vi "波形记录处理.vi"(8 "控件配置文件":string[][](table), 9 "表格":string[][](table)) -> (0 "曲线数量":u16, 2 "曲线名称":string[](array[string]), 3 "波形图":dynamicdata(graph))   [LabVIEW 2021]
uses:
  controls/DataInitDef.ctl
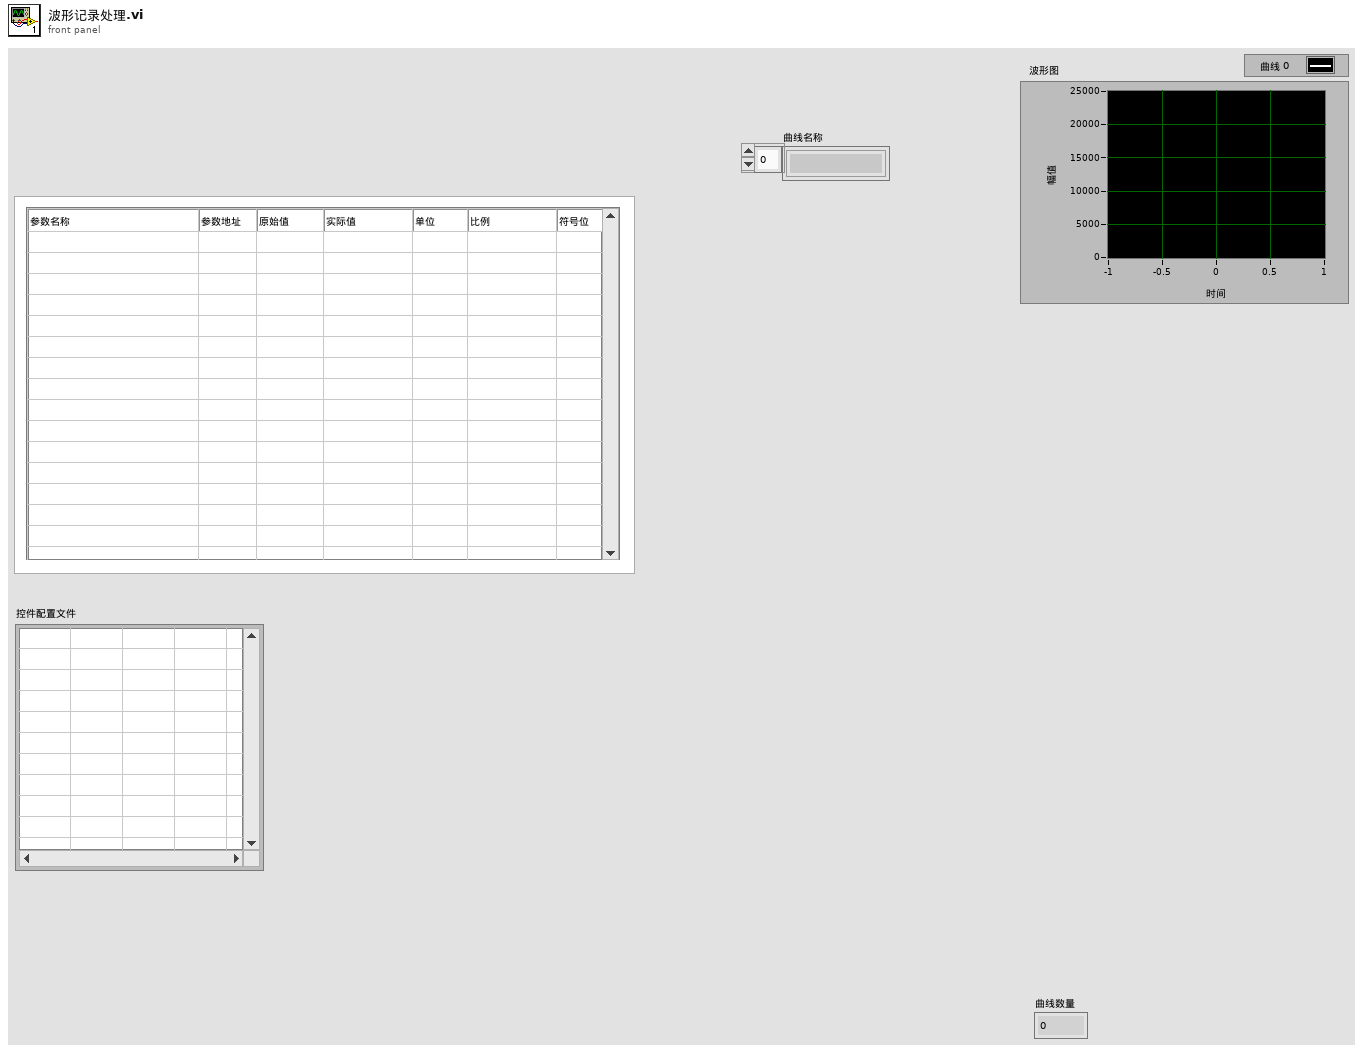
[diagram p1: front panel]
types:
  T1 = typedef "DataInitDef.ctl" = u16
  T2 = cluster{"显示":string, "显示":string, "显示":string, "显示":string, "显示":string, "显示":string, "显示":string, "显示":string, "显示":string, "显示":string, "显示":string, "显示":string, "显示":string, "显示":string, "显示":string, "显示":string}
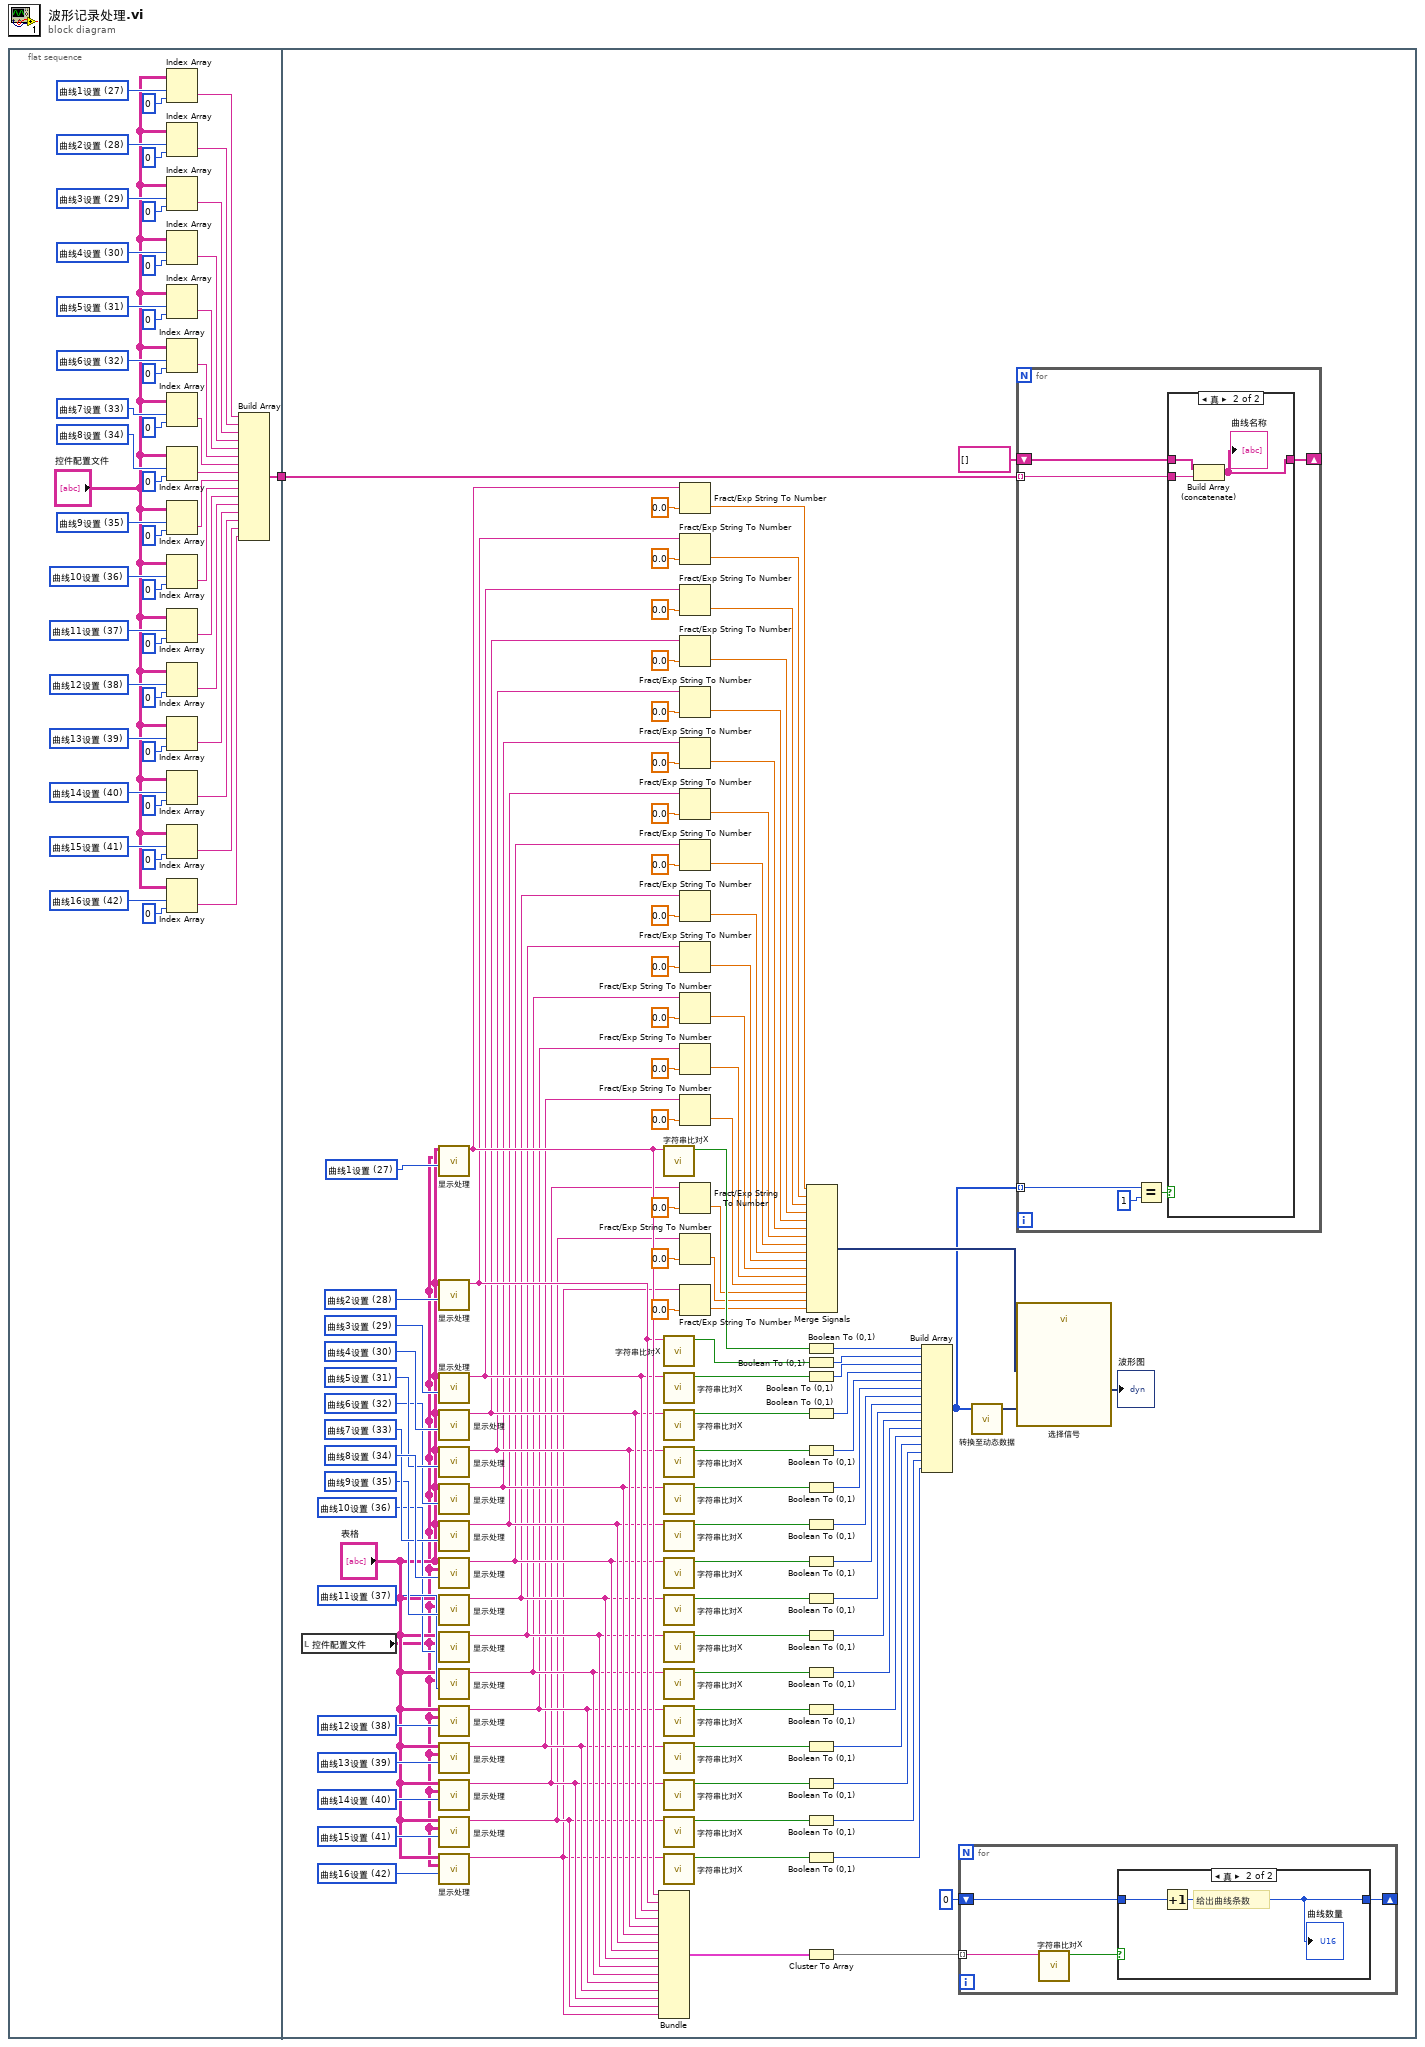
[diagram p0: block diagram]
diagram:
  n1 = flat-sequence {
    tunnel: [w27] -> w1
    tunnel: w1 -> [w115]
    frame #0 {
      w26 = T1 42 items=["刷新间隔", "波特率", "布尔1设置项", "布尔2设置项", "布尔3设置项", "布尔4设置项", "布尔5设置项", "显控1设置", "显控2设置", "显控3设置", "显控4设置", "显控5设置", "显控6设置", "显控7设置", "显控8设置", "显控9设置", "显控10设置", "显控11设置", "显控12设置", "设控1设置", "设控2设置", "设控3设置", "设控4设置", "设控5设置", "设控6设置", "设控7设置", "设控8设置", "曲线1设置", "曲线2设置", "曲线3设置", "曲线4设置", "曲线5设置", "曲线6设置", "曲线7设置", "曲线8设置", "曲线9设置", "曲线10设置", "曲线11设置", "曲线12设置", "曲线13设置", "曲线14设置", "曲线15设置", "曲线16设置", "ID值"] ("DataInitDef")
      w24 = T1 41 items=["刷新间隔", "波特率", "布尔1设置项", "布尔2设置项", "布尔3设置项", "布尔4设置项", "布尔5设置项", "显控1设置", "显控2设置", "显控3设置", "显控4设置", "显控5设置", "显控6设置", "显控7设置", "显控8设置", "显控9设置", "显控10设置", "显控11设置", "显控12设置", "设控1设置", "设控2设置", "设控3设置", "设控4设置", "设控5设置", "设控6设置", "设控7设置", "设控8设置", "曲线1设置", "曲线2设置", "曲线3设置", "曲线4设置", "曲线5设置", "曲线6设置", "曲线7设置", "曲线8设置", "曲线9设置", "曲线10设置", "曲线11设置", "曲线12设置", "曲线13设置", "曲线14设置", "曲线15设置", "曲线16设置", "ID值"] ("DataInitDef")
      w22 = T1 40 items=["刷新间隔", "波特率", "布尔1设置项", "布尔2设置项", "布尔3设置项", "布尔4设置项", "布尔5设置项", "显控1设置", "显控2设置", "显控3设置", "显控4设置", "显控5设置", "显控6设置", "显控7设置", "显控8设置", "显控9设置", "显控10设置", "显控11设置", "显控12设置", "设控1设置", "设控2设置", "设控3设置", "设控4设置", "设控5设置", "设控6设置", "设控7设置", "设控8设置", "曲线1设置", "曲线2设置", "曲线3设置", "曲线4设置", "曲线5设置", "曲线6设置", "曲线7设置", "曲线8设置", "曲线9设置", "曲线10设置", "曲线11设置", "曲线12设置", "曲线13设置", "曲线14设置", "曲线15设置", "曲线16设置", "ID值"] ("DataInitDef")
      w20 = T1 39 items=["刷新间隔", "波特率", "布尔1设置项", "布尔2设置项", "布尔3设置项", "布尔4设置项", "布尔5设置项", "显控1设置", "显控2设置", "显控3设置", "显控4设置", "显控5设置", "显控6设置", "显控7设置", "显控8设置", "显控9设置", "显控10设置", "显控11设置", "显控12设置", "设控1设置", "设控2设置", "设控3设置", "设控4设置", "设控5设置", "设控6设置", "设控7设置", "设控8设置", "曲线1设置", "曲线2设置", "曲线3设置", "曲线4设置", "曲线5设置", "曲线6设置", "曲线7设置", "曲线8设置", "曲线9设置", "曲线10设置", "曲线11设置", "曲线12设置", "曲线13设置", "曲线14设置", "曲线15设置", "曲线16设置", "ID值"] ("DataInitDef")
      w18 = T1 38 items=["刷新间隔", "波特率", "布尔1设置项", "布尔2设置项", "布尔3设置项", "布尔4设置项", "布尔5设置项", "显控1设置", "显控2设置", "显控3设置", "显控4设置", "显控5设置", "显控6设置", "显控7设置", "显控8设置", "显控9设置", "显控10设置", "显控11设置", "显控12设置", "设控1设置", "设控2设置", "设控3设置", "设控4设置", "设控5设置", "设控6设置", "设控7设置", "设控8设置", "曲线1设置", "曲线2设置", "曲线3设置", "曲线4设置", "曲线5设置", "曲线6设置", "曲线7设置", "曲线8设置", "曲线9设置", "曲线10设置", "曲线11设置", "曲线12设置", "曲线13设置", "曲线14设置", "曲线15设置", "曲线16设置", "ID值"] ("DataInitDef")
      w16 = T1 37 items=["刷新间隔", "波特率", "布尔1设置项", "布尔2设置项", "布尔3设置项", "布尔4设置项", "布尔5设置项", "显控1设置", "显控2设置", "显控3设置", "显控4设置", "显控5设置", "显控6设置", "显控7设置", "显控8设置", "显控9设置", "显控10设置", "显控11设置", "显控12设置", "设控1设置", "设控2设置", "设控3设置", "设控4设置", "设控5设置", "设控6设置", "设控7设置", "设控8设置", "曲线1设置", "曲线2设置", "曲线3设置", "曲线4设置", "曲线5设置", "曲线6设置", "曲线7设置", "曲线8设置", "曲线9设置", "曲线10设置", "曲线11设置", "曲线12设置", "曲线13设置", "曲线14设置", "曲线15设置", "曲线16设置", "ID值"] ("DataInitDef")
      w14 = T1 36 items=["刷新间隔", "波特率", "布尔1设置项", "布尔2设置项", "布尔3设置项", "布尔4设置项", "布尔5设置项", "显控1设置", "显控2设置", "显控3设置", "显控4设置", "显控5设置", "显控6设置", "显控7设置", "显控8设置", "显控9设置", "显控10设置", "显控11设置", "显控12设置", "设控1设置", "设控2设置", "设控3设置", "设控4设置", "设控5设置", "设控6设置", "设控7设置", "设控8设置", "曲线1设置", "曲线2设置", "曲线3设置", "曲线4设置", "曲线5设置", "曲线6设置", "曲线7设置", "曲线8设置", "曲线9设置", "曲线10设置", "曲线11设置", "曲线12设置", "曲线13设置", "曲线14设置", "曲线15设置", "曲线16设置", "ID值"] ("DataInitDef")
      w12 = T1 35 items=["刷新间隔", "波特率", "布尔1设置项", "布尔2设置项", "布尔3设置项", "布尔4设置项", "布尔5设置项", "显控1设置", "显控2设置", "显控3设置", "显控4设置", "显控5设置", "显控6设置", "显控7设置", "显控8设置", "显控9设置", "显控10设置", "显控11设置", "显控12设置", "设控1设置", "设控2设置", "设控3设置", "设控4设置", "设控5设置", "设控6设置", "设控7设置", "设控8设置", "曲线1设置", "曲线2设置", "曲线3设置", "曲线4设置", "曲线5设置", "曲线6设置", "曲线7设置", "曲线8设置", "曲线9设置", "曲线10设置", "曲线11设置", "曲线12设置", "曲线13设置", "曲线14设置", "曲线15设置", "曲线16设置", "ID值"] ("DataInitDef")
      w51 = T1 34 items=["刷新间隔", "波特率", "布尔1设置项", "布尔2设置项", "布尔3设置项", "布尔4设置项", "布尔5设置项", "显控1设置", "显控2设置", "显控3设置", "显控4设置", "显控5设置", "显控6设置", "显控7设置", "显控8设置", "显控9设置", "显控10设置", "显控11设置", "显控12设置", "设控1设置", "设控2设置", "设控3设置", "设控4设置", "设控5设置", "设控6设置", "设控7设置", "设控8设置", "曲线1设置", "曲线2设置", "曲线3设置", "曲线4设置", "曲线5设置", "曲线6设置", "曲线7设置", "曲线8设置", "曲线9设置", "曲线10设置", "曲线11设置", "曲线12设置", "曲线13设置", "曲线14设置", "曲线15设置", "曲线16设置", "ID值"] ("DataInitDef")
      w49 = T1 33 items=["刷新间隔", "波特率", "布尔1设置项", "布尔2设置项", "布尔3设置项", "布尔4设置项", "布尔5设置项", "显控1设置", "显控2设置", "显控3设置", "显控4设置", "显控5设置", "显控6设置", "显控7设置", "显控8设置", "显控9设置", "显控10设置", "显控11设置", "显控12设置", "设控1设置", "设控2设置", "设控3设置", "设控4设置", "设控5设置", "设控6设置", "设控7设置", "设控8设置", "曲线1设置", "曲线2设置", "曲线3设置", "曲线4设置", "曲线5设置", "曲线6设置", "曲线7设置", "曲线8设置", "曲线9设置", "曲线10设置", "曲线11设置", "曲线12设置", "曲线13设置", "曲线14设置", "曲线15设置", "曲线16设置", "ID值"] ("DataInitDef")
      w47 = T1 32 items=["刷新间隔", "波特率", "布尔1设置项", "布尔2设置项", "布尔3设置项", "布尔4设置项", "布尔5设置项", "显控1设置", "显控2设置", "显控3设置", "显控4设置", "显控5设置", "显控6设置", "显控7设置", "显控8设置", "显控9设置", "显控10设置", "显控11设置", "显控12设置", "设控1设置", "设控2设置", "设控3设置", "设控4设置", "设控5设置", "设控6设置", "设控7设置", "设控8设置", "曲线1设置", "曲线2设置", "曲线3设置", "曲线4设置", "曲线5设置", "曲线6设置", "曲线7设置", "曲线8设置", "曲线9设置", "曲线10设置", "曲线11设置", "曲线12设置", "曲线13设置", "曲线14设置", "曲线15设置", "曲线16设置", "ID值"] ("DataInitDef")
      w45 = T1 31 items=["刷新间隔", "波特率", "布尔1设置项", "布尔2设置项", "布尔3设置项", "布尔4设置项", "布尔5设置项", "显控1设置", "显控2设置", "显控3设置", "显控4设置", "显控5设置", "显控6设置", "显控7设置", "显控8设置", "显控9设置", "显控10设置", "显控11设置", "显控12设置", "设控1设置", "设控2设置", "设控3设置", "设控4设置", "设控5设置", "设控6设置", "设控7设置", "设控8设置", "曲线1设置", "曲线2设置", "曲线3设置", "曲线4设置", "曲线5设置", "曲线6设置", "曲线7设置", "曲线8设置", "曲线9设置", "曲线10设置", "曲线11设置", "曲线12设置", "曲线13设置", "曲线14设置", "曲线15设置", "曲线16设置", "ID值"] ("DataInitDef")
      w43 = T1 30 items=["刷新间隔", "波特率", "布尔1设置项", "布尔2设置项", "布尔3设置项", "布尔4设置项", "布尔5设置项", "显控1设置", "显控2设置", "显控3设置", "显控4设置", "显控5设置", "显控6设置", "显控7设置", "显控8设置", "显控9设置", "显控10设置", "显控11设置", "显控12设置", "设控1设置", "设控2设置", "设控3设置", "设控4设置", "设控5设置", "设控6设置", "设控7设置", "设控8设置", "曲线1设置", "曲线2设置", "曲线3设置", "曲线4设置", "曲线5设置", "曲线6设置", "曲线7设置", "曲线8设置", "曲线9设置", "曲线10设置", "曲线11设置", "曲线12设置", "曲线13设置", "曲线14设置", "曲线15设置", "曲线16设置", "ID值"] ("DataInitDef")
      w41 = T1 29 items=["刷新间隔", "波特率", "布尔1设置项", "布尔2设置项", "布尔3设置项", "布尔4设置项", "布尔5设置项", "显控1设置", "显控2设置", "显控3设置", "显控4设置", "显控5设置", "显控6设置", "显控7设置", "显控8设置", "显控9设置", "显控10设置", "显控11设置", "显控12设置", "设控1设置", "设控2设置", "设控3设置", "设控4设置", "设控5设置", "设控6设置", "设控7设置", "设控8设置", "曲线1设置", "曲线2设置", "曲线3设置", "曲线4设置", "曲线5设置", "曲线6设置", "曲线7设置", "曲线8设置", "曲线9设置", "曲线10设置", "曲线11设置", "曲线12设置", "曲线13设置", "曲线14设置", "曲线15设置", "曲线16设置", "ID值"] ("DataInitDef")
      w39 = T1 28 items=["刷新间隔", "波特率", "布尔1设置项", "布尔2设置项", "布尔3设置项", "布尔4设置项", "布尔5设置项", "显控1设置", "显控2设置", "显控3设置", "显控4设置", "显控5设置", "显控6设置", "显控7设置", "显控8设置", "显控9设置", "显控10设置", "显控11设置", "显控12设置", "设控1设置", "设控2设置", "设控3设置", "设控4设置", "设控5设置", "设控6设置", "设控7设置", "设控8设置", "曲线1设置", "曲线2设置", "曲线3设置", "曲线4设置", "曲线5设置", "曲线6设置", "曲线7设置", "曲线8设置", "曲线9设置", "曲线10设置", "曲线11设置", "曲线12设置", "曲线13设置", "曲线14设置", "曲线15设置", "曲线16设置", "ID值"] ("DataInitDef")
      w37 = T1 27 items=["刷新间隔", "波特率", "布尔1设置项", "布尔2设置项", "布尔3设置项", "布尔4设置项", "布尔5设置项", "显控1设置", "显控2设置", "显控3设置", "显控4设置", "显控5设置", "显控6设置", "显控7设置", "显控8设置", "显控9设置", "显控10设置", "显控11设置", "显控12设置", "设控1设置", "设控2设置", "设控3设置", "设控4设置", "设控5设置", "设控6设置", "设控7设置", "设控8设置", "曲线1设置", "曲线2设置", "曲线3设置", "曲线4设置", "曲线5设置", "曲线6设置", "曲线7设置", "曲线8设置", "曲线9设置", "曲线10设置", "曲线11设置", "曲线12设置", "曲线13设置", "曲线14设置", "曲线15设置", "曲线16设置", "ID值"] ("DataInitDef")
      n2 = Index Array(array="控件配置文件", index (row)=w37, index (col)=0 ("禁用的索引 (列)")) -> (element=w35:string)
      n3 = Index Array(array="控件配置文件", index (row)=w39, index (col)=0 ("禁用的索引 (列)")) -> (element=w34:string)
      n4 = Index Array(array="控件配置文件", index (row)=w41, index (col)=0 ("禁用的索引 (列)")) -> (element=w33:string)
      n5 = Index Array(array="控件配置文件", index (row)=w43, index (col)=0 ("禁用的索引 (列)")) -> (element=w32:string)
      n6 = Index Array(array="控件配置文件", index (row)=w45, index (col)=0 ("禁用的索引 (列)")) -> (element=w31:string)
      n7 = Index Array(array="控件配置文件", index (row)=w47, index (col)=0 ("禁用的索引 (列)")) -> (element=w30:string)
      n8 = Index Array(array="控件配置文件", index (row)=w49, index (col)=0 ("禁用的索引 (列)")) -> (element=w28:string)
      n9 = Index Array(array="控件配置文件", index (row)=w51, index (col)=0 ("禁用的索引 (列)")) -> (element=w29:string)
      n10 = Index Array(array="控件配置文件", index (row)=w12, index (col)=0 ("禁用的索引 (列)")) -> (element=w9:string)
      n11 = Index Array(array="控件配置文件", index (row)=w14, index (col)=0 ("禁用的索引 (列)")) -> (element=w8:string)
      n12 = Index Array(array="控件配置文件", index (row)=w16, index (col)=0 ("禁用的索引 (列)")) -> (element=w7:string)
      n13 = Index Array(array="控件配置文件", index (row)=w18, index (col)=0 ("禁用的索引 (列)")) -> (element=w6:string)
      n14 = Index Array(array="控件配置文件", index (row)=w20, index (col)=0 ("禁用的索引 (列)")) -> (element=w5:string)
      n15 = Index Array(array="控件配置文件", index (row)=w22, index (col)=0 ("禁用的索引 (列)")) -> (element=w4:string)
      n16 = Index Array(array="控件配置文件", index (row)=w24, index (col)=0 ("禁用的索引 (列)")) -> (element=w3:string)
      n17 = Index Array(array="控件配置文件", index (row)=w26, index (col)=0 ("禁用的索引 (列)")) -> (element=w2:string)
      n18 = Build Array(w35, w34, w33, w32, w31, w30, w28, w29, w9, w8, w7, w6, w5, w4, w3, w2) -> (w27:string[])
    }
    frame #1 {
      w102 = T1 42 items=["刷新间隔", "波特率", "布尔1设置项", "布尔2设置项", "布尔3设置项", "布尔4设置项", "布尔5设置项", "显控1设置", "显控2设置", "显控3设置", "显控4设置", "显控5设置", "显控6设置", "显控7设置", "显控8设置", "显控9设置", "显控10设置", "显控11设置", "显控12设置", "设控1设置", "设控2设置", "设控3设置", "设控4设置", "设控5设置", "设控6设置", "设控7设置", "设控8设置", "曲线1设置", "曲线2设置", "曲线3设置", "曲线4设置", "曲线5设置", "曲线6设置", "曲线7设置", "曲线8设置", "曲线9设置", "曲线10设置", "曲线11设置", "曲线12设置", "曲线13设置", "曲线14设置", "曲线15设置", "曲线16设置", "ID值"] ("DataInitDef")
      w96 = T1 41 items=["刷新间隔", "波特率", "布尔1设置项", "布尔2设置项", "布尔3设置项", "布尔4设置项", "布尔5设置项", "显控1设置", "显控2设置", "显控3设置", "显控4设置", "显控5设置", "显控6设置", "显控7设置", "显控8设置", "显控9设置", "显控10设置", "显控11设置", "显控12设置", "设控1设置", "设控2设置", "设控3设置", "设控4设置", "设控5设置", "设控6设置", "设控7设置", "设控8设置", "曲线1设置", "曲线2设置", "曲线3设置", "曲线4设置", "曲线5设置", "曲线6设置", "曲线7设置", "曲线8设置", "曲线9设置", "曲线10设置", "曲线11设置", "曲线12设置", "曲线13设置", "曲线14设置", "曲线15设置", "曲线16设置", "ID值"] ("DataInitDef")
      w97 = T1 40 items=["刷新间隔", "波特率", "布尔1设置项", "布尔2设置项", "布尔3设置项", "布尔4设置项", "布尔5设置项", "显控1设置", "显控2设置", "显控3设置", "显控4设置", "显控5设置", "显控6设置", "显控7设置", "显控8设置", "显控9设置", "显控10设置", "显控11设置", "显控12设置", "设控1设置", "设控2设置", "设控3设置", "设控4设置", "设控5设置", "设控6设置", "设控7设置", "设控8设置", "曲线1设置", "曲线2设置", "曲线3设置", "曲线4设置", "曲线5设置", "曲线6设置", "曲线7设置", "曲线8设置", "曲线9设置", "曲线10设置", "曲线11设置", "曲线12设置", "曲线13设置", "曲线14设置", "曲线15设置", "曲线16设置", "ID值"] ("DataInitDef")
      w98 = T1 39 items=["刷新间隔", "波特率", "布尔1设置项", "布尔2设置项", "布尔3设置项", "布尔4设置项", "布尔5设置项", "显控1设置", "显控2设置", "显控3设置", "显控4设置", "显控5设置", "显控6设置", "显控7设置", "显控8设置", "显控9设置", "显控10设置", "显控11设置", "显控12设置", "设控1设置", "设控2设置", "设控3设置", "设控4设置", "设控5设置", "设控6设置", "设控7设置", "设控8设置", "曲线1设置", "曲线2设置", "曲线3设置", "曲线4设置", "曲线5设置", "曲线6设置", "曲线7设置", "曲线8设置", "曲线9设置", "曲线10设置", "曲线11设置", "曲线12设置", "曲线13设置", "曲线14设置", "曲线15设置", "曲线16设置", "ID值"] ("DataInitDef")
      w99 = T1 38 items=["刷新间隔", "波特率", "布尔1设置项", "布尔2设置项", "布尔3设置项", "布尔4设置项", "布尔5设置项", "显控1设置", "显控2设置", "显控3设置", "显控4设置", "显控5设置", "显控6设置", "显控7设置", "显控8设置", "显控9设置", "显控10设置", "显控11设置", "显控12设置", "设控1设置", "设控2设置", "设控3设置", "设控4设置", "设控5设置", "设控6设置", "设控7设置", "设控8设置", "曲线1设置", "曲线2设置", "曲线3设置", "曲线4设置", "曲线5设置", "曲线6设置", "曲线7设置", "曲线8设置", "曲线9设置", "曲线10设置", "曲线11设置", "曲线12设置", "曲线13设置", "曲线14设置", "曲线15设置", "曲线16设置", "ID值"] ("DataInitDef")
      w101 = T1 37 items=["刷新间隔", "波特率", "布尔1设置项", "布尔2设置项", "布尔3设置项", "布尔4设置项", "布尔5设置项", "显控1设置", "显控2设置", "显控3设置", "显控4设置", "显控5设置", "显控6设置", "显控7设置", "显控8设置", "显控9设置", "显控10设置", "显控11设置", "显控12设置", "设控1设置", "设控2设置", "设控3设置", "设控4设置", "设控5设置", "设控6设置", "设控7设置", "设控8设置", "曲线1设置", "曲线2设置", "曲线3设置", "曲线4设置", "曲线5设置", "曲线6设置", "曲线7设置", "曲线8设置", "曲线9设置", "曲线10设置", "曲线11设置", "曲线12设置", "曲线13设置", "曲线14设置", "曲线15设置", "曲线16设置", "ID值"] ("DataInitDef")
      w100 = T1 36 items=["刷新间隔", "波特率", "布尔1设置项", "布尔2设置项", "布尔3设置项", "布尔4设置项", "布尔5设置项", "显控1设置", "显控2设置", "显控3设置", "显控4设置", "显控5设置", "显控6设置", "显控7设置", "显控8设置", "显控9设置", "显控10设置", "显控11设置", "显控12设置", "设控1设置", "设控2设置", "设控3设置", "设控4设置", "设控5设置", "设控6设置", "设控7设置", "设控8设置", "曲线1设置", "曲线2设置", "曲线3设置", "曲线4设置", "曲线5设置", "曲线6设置", "曲线7设置", "曲线8设置", "曲线9设置", "曲线10设置", "曲线11设置", "曲线12设置", "曲线13设置", "曲线14设置", "曲线15设置", "曲线16设置", "ID值"] ("DataInitDef")
      w103 = T1 35 items=["刷新间隔", "波特率", "布尔1设置项", "布尔2设置项", "布尔3设置项", "布尔4设置项", "布尔5设置项", "显控1设置", "显控2设置", "显控3设置", "显控4设置", "显控5设置", "显控6设置", "显控7设置", "显控8设置", "显控9设置", "显控10设置", "显控11设置", "显控12设置", "设控1设置", "设控2设置", "设控3设置", "设控4设置", "设控5设置", "设控6设置", "设控7设置", "设控8设置", "曲线1设置", "曲线2设置", "曲线3设置", "曲线4设置", "曲线5设置", "曲线6设置", "曲线7设置", "曲线8设置", "曲线9设置", "曲线10设置", "曲线11设置", "曲线12设置", "曲线13设置", "曲线14设置", "曲线15设置", "曲线16设置", "ID值"] ("DataInitDef")
      w148 = T1 34 items=["刷新间隔", "波特率", "布尔1设置项", "布尔2设置项", "布尔3设置项", "布尔4设置项", "布尔5设置项", "显控1设置", "显控2设置", "显控3设置", "显控4设置", "显控5设置", "显控6设置", "显控7设置", "显控8设置", "显控9设置", "显控10设置", "显控11设置", "显控12设置", "设控1设置", "设控2设置", "设控3设置", "设控4设置", "设控5设置", "设控6设置", "设控7设置", "设控8设置", "曲线1设置", "曲线2设置", "曲线3设置", "曲线4设置", "曲线5设置", "曲线6设置", "曲线7设置", "曲线8设置", "曲线9设置", "曲线10设置", "曲线11设置", "曲线12设置", "曲线13设置", "曲线14设置", "曲线15设置", "曲线16设置", "ID值"] ("DataInitDef")
      w142 = T1 33 items=["刷新间隔", "波特率", "布尔1设置项", "布尔2设置项", "布尔3设置项", "布尔4设置项", "布尔5设置项", "显控1设置", "显控2设置", "显控3设置", "显控4设置", "显控5设置", "显控6设置", "显控7设置", "显控8设置", "显控9设置", "显控10设置", "显控11设置", "显控12设置", "设控1设置", "设控2设置", "设控3设置", "设控4设置", "设控5设置", "设控6设置", "设控7设置", "设控8设置", "曲线1设置", "曲线2设置", "曲线3设置", "曲线4设置", "曲线5设置", "曲线6设置", "曲线7设置", "曲线8设置", "曲线9设置", "曲线10设置", "曲线11设置", "曲线12设置", "曲线13设置", "曲线14设置", "曲线15设置", "曲线16设置", "ID值"] ("DataInitDef")
      w143 = T1 32 items=["刷新间隔", "波特率", "布尔1设置项", "布尔2设置项", "布尔3设置项", "布尔4设置项", "布尔5设置项", "显控1设置", "显控2设置", "显控3设置", "显控4设置", "显控5设置", "显控6设置", "显控7设置", "显控8设置", "显控9设置", "显控10设置", "显控11设置", "显控12设置", "设控1设置", "设控2设置", "设控3设置", "设控4设置", "设控5设置", "设控6设置", "设控7设置", "设控8设置", "曲线1设置", "曲线2设置", "曲线3设置", "曲线4设置", "曲线5设置", "曲线6设置", "曲线7设置", "曲线8设置", "曲线9设置", "曲线10设置", "曲线11设置", "曲线12设置", "曲线13设置", "曲线14设置", "曲线15设置", "曲线16设置", "ID值"] ("DataInitDef")
      w144 = T1 31 items=["刷新间隔", "波特率", "布尔1设置项", "布尔2设置项", "布尔3设置项", "布尔4设置项", "布尔5设置项", "显控1设置", "显控2设置", "显控3设置", "显控4设置", "显控5设置", "显控6设置", "显控7设置", "显控8设置", "显控9设置", "显控10设置", "显控11设置", "显控12设置", "设控1设置", "设控2设置", "设控3设置", "设控4设置", "设控5设置", "设控6设置", "设控7设置", "设控8设置", "曲线1设置", "曲线2设置", "曲线3设置", "曲线4设置", "曲线5设置", "曲线6设置", "曲线7设置", "曲线8设置", "曲线9设置", "曲线10设置", "曲线11设置", "曲线12设置", "曲线13设置", "曲线14设置", "曲线15设置", "曲线16设置", "ID值"] ("DataInitDef")
      w145 = T1 30 items=["刷新间隔", "波特率", "布尔1设置项", "布尔2设置项", "布尔3设置项", "布尔4设置项", "布尔5设置项", "显控1设置", "显控2设置", "显控3设置", "显控4设置", "显控5设置", "显控6设置", "显控7设置", "显控8设置", "显控9设置", "显控10设置", "显控11设置", "显控12设置", "设控1设置", "设控2设置", "设控3设置", "设控4设置", "设控5设置", "设控6设置", "设控7设置", "设控8设置", "曲线1设置", "曲线2设置", "曲线3设置", "曲线4设置", "曲线5设置", "曲线6设置", "曲线7设置", "曲线8设置", "曲线9设置", "曲线10设置", "曲线11设置", "曲线12设置", "曲线13设置", "曲线14设置", "曲线15设置", "曲线16设置", "ID值"] ("DataInitDef")
      w147 = T1 29 items=["刷新间隔", "波特率", "布尔1设置项", "布尔2设置项", "布尔3设置项", "布尔4设置项", "布尔5设置项", "显控1设置", "显控2设置", "显控3设置", "显控4设置", "显控5设置", "显控6设置", "显控7设置", "显控8设置", "显控9设置", "显控10设置", "显控11设置", "显控12设置", "设控1设置", "设控2设置", "设控3设置", "设控4设置", "设控5设置", "设控6设置", "设控7设置", "设控8设置", "曲线1设置", "曲线2设置", "曲线3设置", "曲线4设置", "曲线5设置", "曲线6设置", "曲线7设置", "曲线8设置", "曲线9设置", "曲线10设置", "曲线11设置", "曲线12设置", "曲线13设置", "曲线14设置", "曲线15设置", "曲线16设置", "ID值"] ("DataInitDef")
      w146 = T1 28 items=["刷新间隔", "波特率", "布尔1设置项", "布尔2设置项", "布尔3设置项", "布尔4设置项", "布尔5设置项", "显控1设置", "显控2设置", "显控3设置", "显控4设置", "显控5设置", "显控6设置", "显控7设置", "显控8设置", "显控9设置", "显控10设置", "显控11设置", "显控12设置", "设控1设置", "设控2设置", "设控3设置", "设控4设置", "设控5设置", "设控6设置", "设控7设置", "设控8设置", "曲线1设置", "曲线2设置", "曲线3设置", "曲线4设置", "曲线5设置", "曲线6设置", "曲线7设置", "曲线8设置", "曲线9设置", "曲线10设置", "曲线11设置", "曲线12设置", "曲线13设置", "曲线14设置", "曲线15设置", "曲线16设置", "ID值"] ("DataInitDef")
      w149 = T1 27 items=["刷新间隔", "波特率", "布尔1设置项", "布尔2设置项", "布尔3设置项", "布尔4设置项", "布尔5设置项", "显控1设置", "显控2设置", "显控3设置", "显控4设置", "显控5设置", "显控6设置", "显控7设置", "显控8设置", "显控9设置", "显控10设置", "显控11设置", "显控12设置", "设控1设置", "设控2设置", "设控3设置", "设控4设置", "设控5设置", "设控6设置", "设控7设置", "设控8设置", "曲线1设置", "曲线2设置", "曲线3设置", "曲线4设置", "曲线5设置", "曲线6设置", "曲线7设置", "曲线8设置", "曲线9设置", "曲线10设置", "曲线11设置", "曲线12设置", "曲线13设置", "曲线14设置", "曲线15设置", "曲线16设置", "ID值"] ("DataInitDef")
      n19 = local read "控件配置文件"() -> (w94:string[][])
      n20 = call "显示处理.vi"("项目"=w149, "配置文件"=w94, "表格"="表格") -> ("显示"=w139:string)  [unwired: 8 in]
      n21 = call "显示处理.vi"("项目"=w146, "配置文件"=w94, "表格"="表格") -> ("显示"=w138:string)  [unwired: 8 in]
      n22 = call "显示处理.vi"("项目"=w147, "配置文件"=w94, "表格"="表格") -> ("显示"=w137:string)  [unwired: 8 in]
      n23 = call "显示处理.vi"("项目"=w145, "配置文件"=w94, "表格"="表格") -> ("显示"=w136:string)  [unwired: 8 in]
      n24 = call "显示处理.vi"("项目"=w144, "配置文件"=w94, "表格"="表格") -> ("显示"=w135:string)  [unwired: 8 in]
      n25 = call "显示处理.vi"("项目"=w143, "配置文件"=w94, "表格"="表格") -> ("显示"=w134:string)  [unwired: 8 in]
      n26 = call "显示处理.vi"("项目"=w142, "配置文件"=w94, "表格"="表格") -> ("显示"=w105:string)  [unwired: 8 in]
      n27 = call "显示处理.vi"("项目"=w148, "配置文件"=w94, "表格"="表格") -> ("显示"=w104:string)  [unwired: 8 in]
      n28 = call "显示处理.vi"("项目"=w103, "配置文件"=w94, "表格"="表格") -> ("显示"=w61:string)  [unwired: 8 in]
      n29 = call "显示处理.vi"("项目"=w100, "配置文件"=w94, "表格"="表格") -> ("显示"=w60:string)  [unwired: 8 in]
      n30 = call "显示处理.vi"("项目"=w101, "配置文件"=w94, "表格"="表格") -> ("显示"=w59:string)  [unwired: 8 in]
      n31 = call "显示处理.vi"("项目"=w99, "配置文件"=w94, "表格"="表格") -> ("显示"=w58:string)  [unwired: 8 in]
      n32 = call "显示处理.vi"("项目"=w98, "配置文件"=w94, "表格"="表格") -> ("显示"=w57:string)  [unwired: 8 in]
      n33 = call "显示处理.vi"("项目"=w97, "配置文件"=w94, "表格"="表格") -> ("显示"=w56:string)  [unwired: 8 in]
      n34 = call "显示处理.vi"("项目"=w96, "配置文件"=w94, "表格"="表格") -> ("显示"=w55:string)  [unwired: 8 in]
      n35 = call "显示处理.vi"("项目"=w102, "配置文件"=w94, "表格"="表格") -> ("显示"=w54:string)  [unwired: 8 in]
      n36 = Bundle("显示"=w139, "显示"=w138, "显示"=w137, "显示"=w136, "显示"=w135, "显示"=w134, "显示"=w105, "显示"=w104, "显示"=w61, "显示"=w60, "显示"=w59, "显示"=w58, "显示"=w57, "显示"=w56, "显示"=w55, "显示"=w54) -> (w53:T2)  [unwired: 1 in]
      n37 = call "字符串比对X.vi"("字符串"=w139) -> ("布尔"=w133:bool)  [unwired: 10 in]
      n38 = call "字符串比对X.vi"("字符串"=w138) -> ("布尔"=w132:bool)  [unwired: 10 in]
      n39 = call "字符串比对X.vi"("字符串"=w137) -> ("布尔"=w131:bool)  [unwired: 10 in]
      n40 = call "字符串比对X.vi"("字符串"=w136) -> ("布尔"=w130:bool)  [unwired: 10 in]
      n41 = call "字符串比对X.vi"("字符串"=w135) -> ("布尔"=w129:bool)  [unwired: 10 in]
      n42 = call "字符串比对X.vi"("字符串"=w134) -> ("布尔"=w128:bool)  [unwired: 10 in]
      n43 = call "字符串比对X.vi"("字符串"=w105) -> ("布尔"=w127:bool)  [unwired: 10 in]
      n44 = call "字符串比对X.vi"("字符串"=w104) -> ("布尔"=w126:bool)  [unwired: 10 in]
      n45 = call "字符串比对X.vi"("字符串"=w61) -> ("布尔"=w77:bool)  [unwired: 10 in]
      n46 = call "字符串比对X.vi"("字符串"=w60) -> ("布尔"=w76:bool)  [unwired: 10 in]
      n47 = call "字符串比对X.vi"("字符串"=w59) -> ("布尔"=w75:bool)  [unwired: 10 in]
      n48 = call "字符串比对X.vi"("字符串"=w58) -> ("布尔"=w74:bool)  [unwired: 10 in]
      n49 = call "字符串比对X.vi"("字符串"=w57) -> ("布尔"=w73:bool)  [unwired: 10 in]
      n50 = call "字符串比对X.vi"("字符串"=w56) -> ("布尔"=w72:bool)  [unwired: 10 in]
      n51 = call "字符串比对X.vi"("字符串"=w55) -> ("布尔"=w71:bool)  [unwired: 10 in]
      n52 = call "字符串比对X.vi"("字符串"=w54) -> ("布尔"=w70:bool)  [unwired: 10 in]
      n53 = Fract/Exp String To Number(string=w139, default (0 dbl)=0.0 ("默认(0 DBL)")) -> (number=w151:dbl)  [unwired: 2 in, 1 out]
      n54 = Fract/Exp String To Number(string=w138, default (0 dbl)=0.0 ("默认(0 DBL)")) -> (number=w152:dbl)  [unwired: 2 in, 1 out]
      n55 = Fract/Exp String To Number(string=w137, default (0 dbl)=0.0 ("默认(0 DBL)")) -> (number=w153:dbl)  [unwired: 2 in, 1 out]
      n56 = Fract/Exp String To Number(string=w136, default (0 dbl)=0.0 ("默认(0 DBL)")) -> (number=w154:dbl)  [unwired: 2 in, 1 out]
      n57 = Fract/Exp String To Number(string=w135, default (0 dbl)=0.0 ("默认(0 DBL)")) -> (number=w155:dbl)  [unwired: 2 in, 1 out]
      n58 = Fract/Exp String To Number(string=w134, default (0 dbl)=0.0 ("默认(0 DBL)")) -> (number=w156:dbl)  [unwired: 2 in, 1 out]
      n59 = Fract/Exp String To Number(string=w105, default (0 dbl)=0.0 ("默认(0 DBL)")) -> (number=w157:dbl)  [unwired: 2 in, 1 out]
      n60 = Fract/Exp String To Number(string=w104, default (0 dbl)=0.0 ("默认(0 DBL)")) -> (number=w158:dbl)  [unwired: 2 in, 1 out]
      n61 = Fract/Exp String To Number(string=w61, default (0 dbl)=0.0 ("默认(0 DBL)")) -> (number=w85:dbl)  [unwired: 2 in, 1 out]
      n62 = Fract/Exp String To Number(string=w60, default (0 dbl)=0.0 ("默认(0 DBL)")) -> (number=w84:dbl)  [unwired: 2 in, 1 out]
      n63 = Fract/Exp String To Number(string=w59, default (0 dbl)=0.0 ("默认(0 DBL)")) -> (number=w83:dbl)  [unwired: 2 in, 1 out]
      n64 = Fract/Exp String To Number(string=w58, default (0 dbl)=0.0 ("默认(0 DBL)")) -> (number=w82:dbl)  [unwired: 2 in, 1 out]
      n65 = Fract/Exp String To Number(string=w57, default (0 dbl)=0.0 ("默认(0 DBL)")) -> (number=w81:dbl)  [unwired: 2 in, 1 out]
      n66 = Fract/Exp String To Number(string=w56, default (0 dbl)=0.0 ("默认(0 DBL)")) -> (number=w80:dbl)  [unwired: 2 in, 1 out]
      n67 = Fract/Exp String To Number(string=w55, default (0 dbl)=0.0 ("默认(0 DBL)")) -> (number=w79:dbl)  [unwired: 2 in, 1 out]
      n68 = Fract/Exp String To Number(string=w54, default (0 dbl)=0.0 ("默认(0 DBL)")) -> (number=w78:dbl)  [unwired: 2 in, 1 out]
      n69 = Boolean To (0,1)(Boolean=w133) -> (0, 1=w125:i16)
      n70 = Boolean To (0,1)(Boolean=w132) -> (0, 1=w124:i16)
      n71 = Boolean To (0,1)(Boolean=w131) -> (0, 1=w123:i16)
      n72 = Boolean To (0,1)(Boolean=w130) -> (0, 1=w122:i16)
      n73 = Boolean To (0,1)(Boolean=w129) -> (0, 1=w121:i16)
      n74 = Boolean To (0,1)(Boolean=w128) -> (0, 1=w120:i16)
      n75 = Boolean To (0,1)(Boolean=w127) -> (0, 1=w119:i16)
      n76 = Boolean To (0,1)(Boolean=w126) -> (0, 1=w118:i16)
      n77 = Boolean To (0,1)(Boolean=w77) -> (0, 1=w69:i16)
      n78 = Boolean To (0,1)(Boolean=w76) -> (0, 1=w68:i16)
      n79 = Boolean To (0,1)(Boolean=w75) -> (0, 1=w67:i16)
      n80 = Boolean To (0,1)(Boolean=w74) -> (0, 1=w66:i16)
      n81 = Boolean To (0,1)(Boolean=w73) -> (0, 1=w65:i16)
      n82 = Boolean To (0,1)(Boolean=w72) -> (0, 1=w64:i16)
      n83 = Boolean To (0,1)(Boolean=w71) -> (0, 1=w63:i16)
      n84 = Boolean To (0,1)(Boolean=w70) -> (0, 1=w62:i16)
      n85 = Cluster To Array(cluster=w53) -> (array=w52:string[])
      n86 = Merge Signals(w151, w152, w153, w154, w155, w156, w157, w158, w85, w84, w83, w82, w81, w80, w79, w78) -> (w140:dynamicdata)
      n87 = Build Array(w125, w124, w123, w122, w121, w120, w119, w118, w69, w68, w67, w66, w65, w64, w63, w62) -> (w116:i16[])
      n88 = for {
        shift-right: [w171] -> _
        shift-left: u16 0 -> [w170]
        tunnel: w52 -> [w169] mode=indexing
        n89 = call "字符串比对X.vi"("字符串"=w169) -> ("布尔"=w172:bool)  [unwired: 10 in]
        n90 = case shown="真" w172 {
          tunnel: [w173 w175] -> w171
          tunnel: w170 -> [w173 w174]
          frame False {
          }
          frame True {
            # "给出曲线条数"
            n91 = Increment ("加1")(x=w174) -> (x+1=w175:u16)
            "曲线数量" <- w175
          }
        }
      }
      n92 = call "转换至动态数据"("Array"=w116) -> ("Dynamic Data Type"=w141:dynamicdata)  [unwired: 3 in]
      n93 = for {
        tunnel: w116 -> [w164] mode=indexing
        shift-right: [w161] -> _
        shift-left: string[] [] -> [w160]
        tunnel: w115 -> [w159] mode=indexing
        n94 = Equal?(x=w164, y=i16 1) -> (x = y?=w162:bool)
        n95 = case shown="真" w162 {
          tunnel: [w165 w166] -> w161
          tunnel: w160 -> [w165 w168]
          tunnel: w159 -> [_ w167]
          frame False {
          }
          frame True {
            n96 = Build Array (concatenate)(w168, w167) -> (w166:string[])
            "曲线名称" <- w166
          }
        }
      }
      n97 = call "选择信号"("Selector Input"=w141, "Signals"=w140) -> ("Signal Out"=→"波形图":dynamicdata)  [unwired: 8 in, 1 out]
    }
  }
